vi "Pade_mn(x).vi"(9 "x":dbl, 10 "denominator":dbl[](array[numeric])=[1.0, 0.0, 0.0367101138426, 0.0, 0.0006886010743, 0.0, 7.2619287682809e-06], 11 "numerator":dbl[](array[numeric])=[0.0, 1.0, 0.0, -0.129957, 0.0, 0.0029035821005]) -> (3 "Pm/n (x)":dbl)   [LabVIEW 2020]
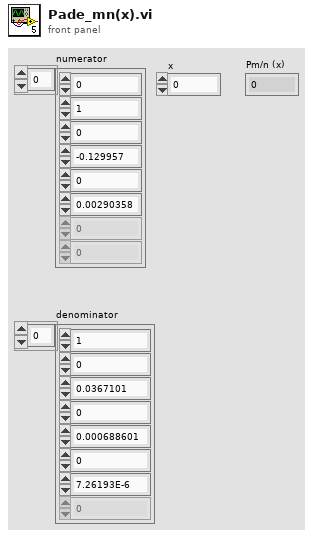
[diagram p1: front panel]
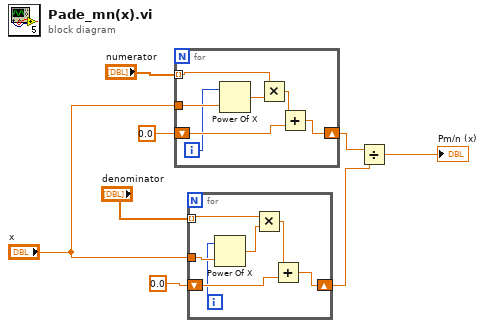
[diagram p0: block diagram]
diagram:
  n1 = for {
    tunnel: "x" -> [w15]
    tunnel: "numerator" -> [w11] mode=indexing
    shift-right: [w14] -> w6
    shift-left: 0.0 -> [w13]
    i -> [w9]
    n2 = Power Of X(1:w15, 2:w9) -> (0:w12:dbl)
    n3 = Multiply(x=w11, y=w12) -> (x*y=w10:dbl)
    n4 = Add(x=w10, y=w13) -> (x+y=w14:dbl)
  }
  n5 = for {
    tunnel: "x" -> [w22]
    tunnel: "denominator" -> [w19] mode=indexing
    shift-right: [w21] -> w7
    shift-left: 0.0 -> [w20]
    i -> [w16]
    n6 = Power Of X(1:w22, 2:w16) -> (0:w18:dbl)
    n7 = Multiply(x=w19, y=w18) -> (x*y=w17:dbl)
    n8 = Add(x=w17, y=w20) -> (x+y=w21:dbl)
  }
  n9 = Divide(x=w6, y=w7) -> (x/y=→"Pm/n (x)":dbl)
